vi "Clapp Oscilator Calcuator.vi"() -> ()   [LabVIEW 2013]
panel:
  in  "L Units":enum16{"H", "mH", "µH", "nH", "pH"}(ring)
  out "L (Actual)":dbl format="%#_6e"
  in  "L":dbl
  in  "C2 Units":enum16{"F", "mF", "µF", "nF", "pF"}(ring)
  in  "C1 Units":enum16{"F", "mF", "µF", "nF", "pF"}(ring)
  in  "C0 Units":enum16{"F", "mF", "µF", "nF", "pF"}(ring)
  out "C3 (Actual)":dbl format="%#_6e"
  out "C1 (Actual)":dbl format="%#_6e"
  out "C0 (Actual)":dbl format="%#_6e"
  in  "C2":dbl
  in  "C1":dbl
  in  "C0":dbl
  out "Frequency":dbl format="%#_g Hz"
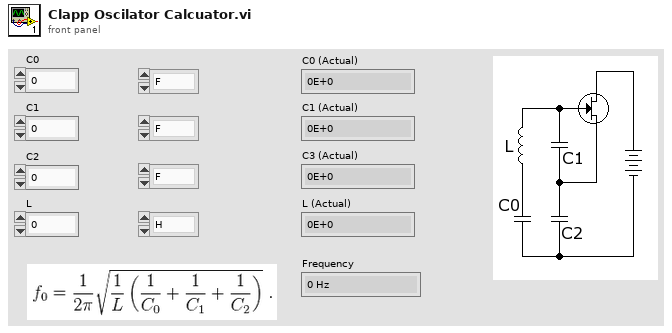
[diagram p1: front panel]
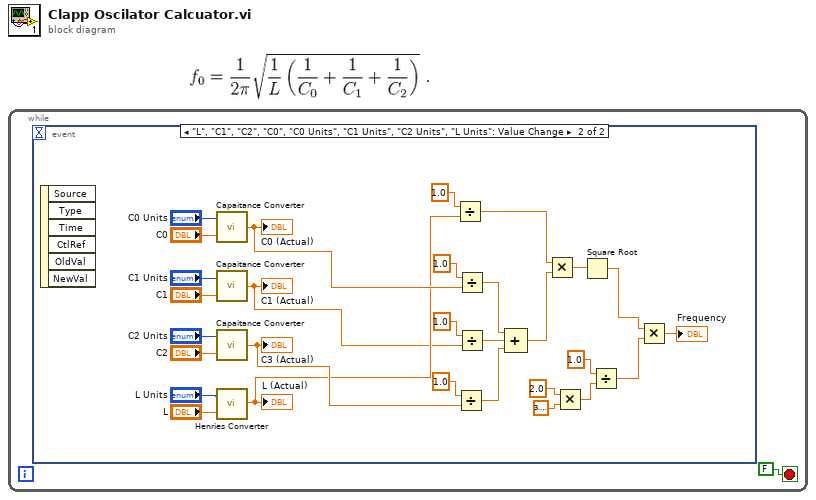
[diagram p0: block diagram]
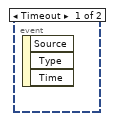
[diagram p2: hidden frame]
diagram:
  n1 = while {
    stop <- FALSE stop-if-true
    n2 = event shown="[1] \"L\", \"C1\", \"C2\", \"C0\", \"C0 Units\", \"C1 Units\", \"C2 Units\", \"L Units\": Value Change" {
      selector: _ -> [_ _]
      dyn-events: _ -> [_ _]
      timeout: _ -> [_ _]
      event Timeout {
        n3 = event-data() -> ()  [unwired: 1 in, 3 out]
      }
      event "L", "C1", "C2", "C0", "C0 Units", "C1 Units", "C2 Units", "L Units": Value Change {
        n4 = event-data() -> ()  [unwired: 1 in, 6 out]
        n5 = call "Capaitance Converter.vi"("C in"="C0", "C Units"="C0 Units") -> ("C out"=w5:dbl)
        "C0 (Actual)" <- w5
        n6 = call "Capaitance Converter.vi"("C in"="C1", "C Units"="C1 Units") -> ("C out"=w2:dbl)
        "C1 (Actual)" <- w2
        n7 = call "Capaitance Converter.vi"("C in"="C2", "C Units"="C2 Units") -> ("C out"=w4:dbl)
        "C3 (Actual)" <- w4
        n8 = call "Henries Converter.vi"("L in"="L", "L Units"="L Units") -> ("L out"=w3:dbl)
        "L (Actual)" <- w3
        n9 = Divide(x=1.0, y=w3) -> (x/y=w18:dbl)
        n10 = Divide(x=1.0, y=w4) -> (x/y=w21:dbl)
        n11 = Divide(x=1.0, y=w5) -> (x/y=w22:dbl)
        n12 = Divide(x=1.0, y=w2) -> (x/y=w23:dbl)
        n13 = Compound Arithmetic op=ADD(w22, w23, w21) -> (w19:dbl)
        n14 = Multiply(x=w18, y=w19) -> (x*y=w17:dbl)
        n15 = Multiply(x=2.0, y=3.141592653589793) -> (x*y=w28:dbl)
        n16 = Square Root(x=w17) -> (sqrt(x)=w15:dbl)
        n17 = Divide(x=1.0, y=w28) -> (x/y=w16:dbl)
        n18 = Multiply(x=w15, y=w16) -> (x*y=→"Frequency":dbl)
      }
    }
  }
